vi "系统设置全局变量.vi"() -> ()   [LabVIEW 2016]
panel:
  in  "多参数运行间隔":i16=4 min=0 max=24
  in  "电源串口":refnum<visa-resource-name>
  out "流程测试中":bool
  out "24H周期设置":bool[](array[boolean])
  out "启用运维打卡":bool caption="启用"
  in  "权限密码":u32[](array[numeric])=[0, 23506, 783523506, 783523103]
  in  "站点系列号":string
  in  "系统重启设置":T1 {"分" max=59 format="%02.0f"; "时" max=23 format="%02.0f"}
  in  "首页显示信息设置":T2={"水温"=TRUE, "pH"=FALSE, "DO"=FALSE, "Cond"=FALSE, "Turb"=FALSE, "氨氮"=FALSE, "总磷"=FALSE, "总氮"=FALSE, "CODMn"=FALSE, "CODCr"=FALSE, "水位"=FALSE, "流速"=FALSE, "瞬时流量"=FALSE, "ORP"=FALSE, "氟化物"=FALSE, "铅"=FALSE, "镉"=FALSE, "铜"=FALSE, "锌"=FALSE, "汞"=FALSE, "叶绿素a"=FALSE, "藻密度"=FALSE, "氯化物"=FALSE, "挥发酚"=FALSE, "盐度"=FALSE}
  # "频次："
  # "时间："
  # "："
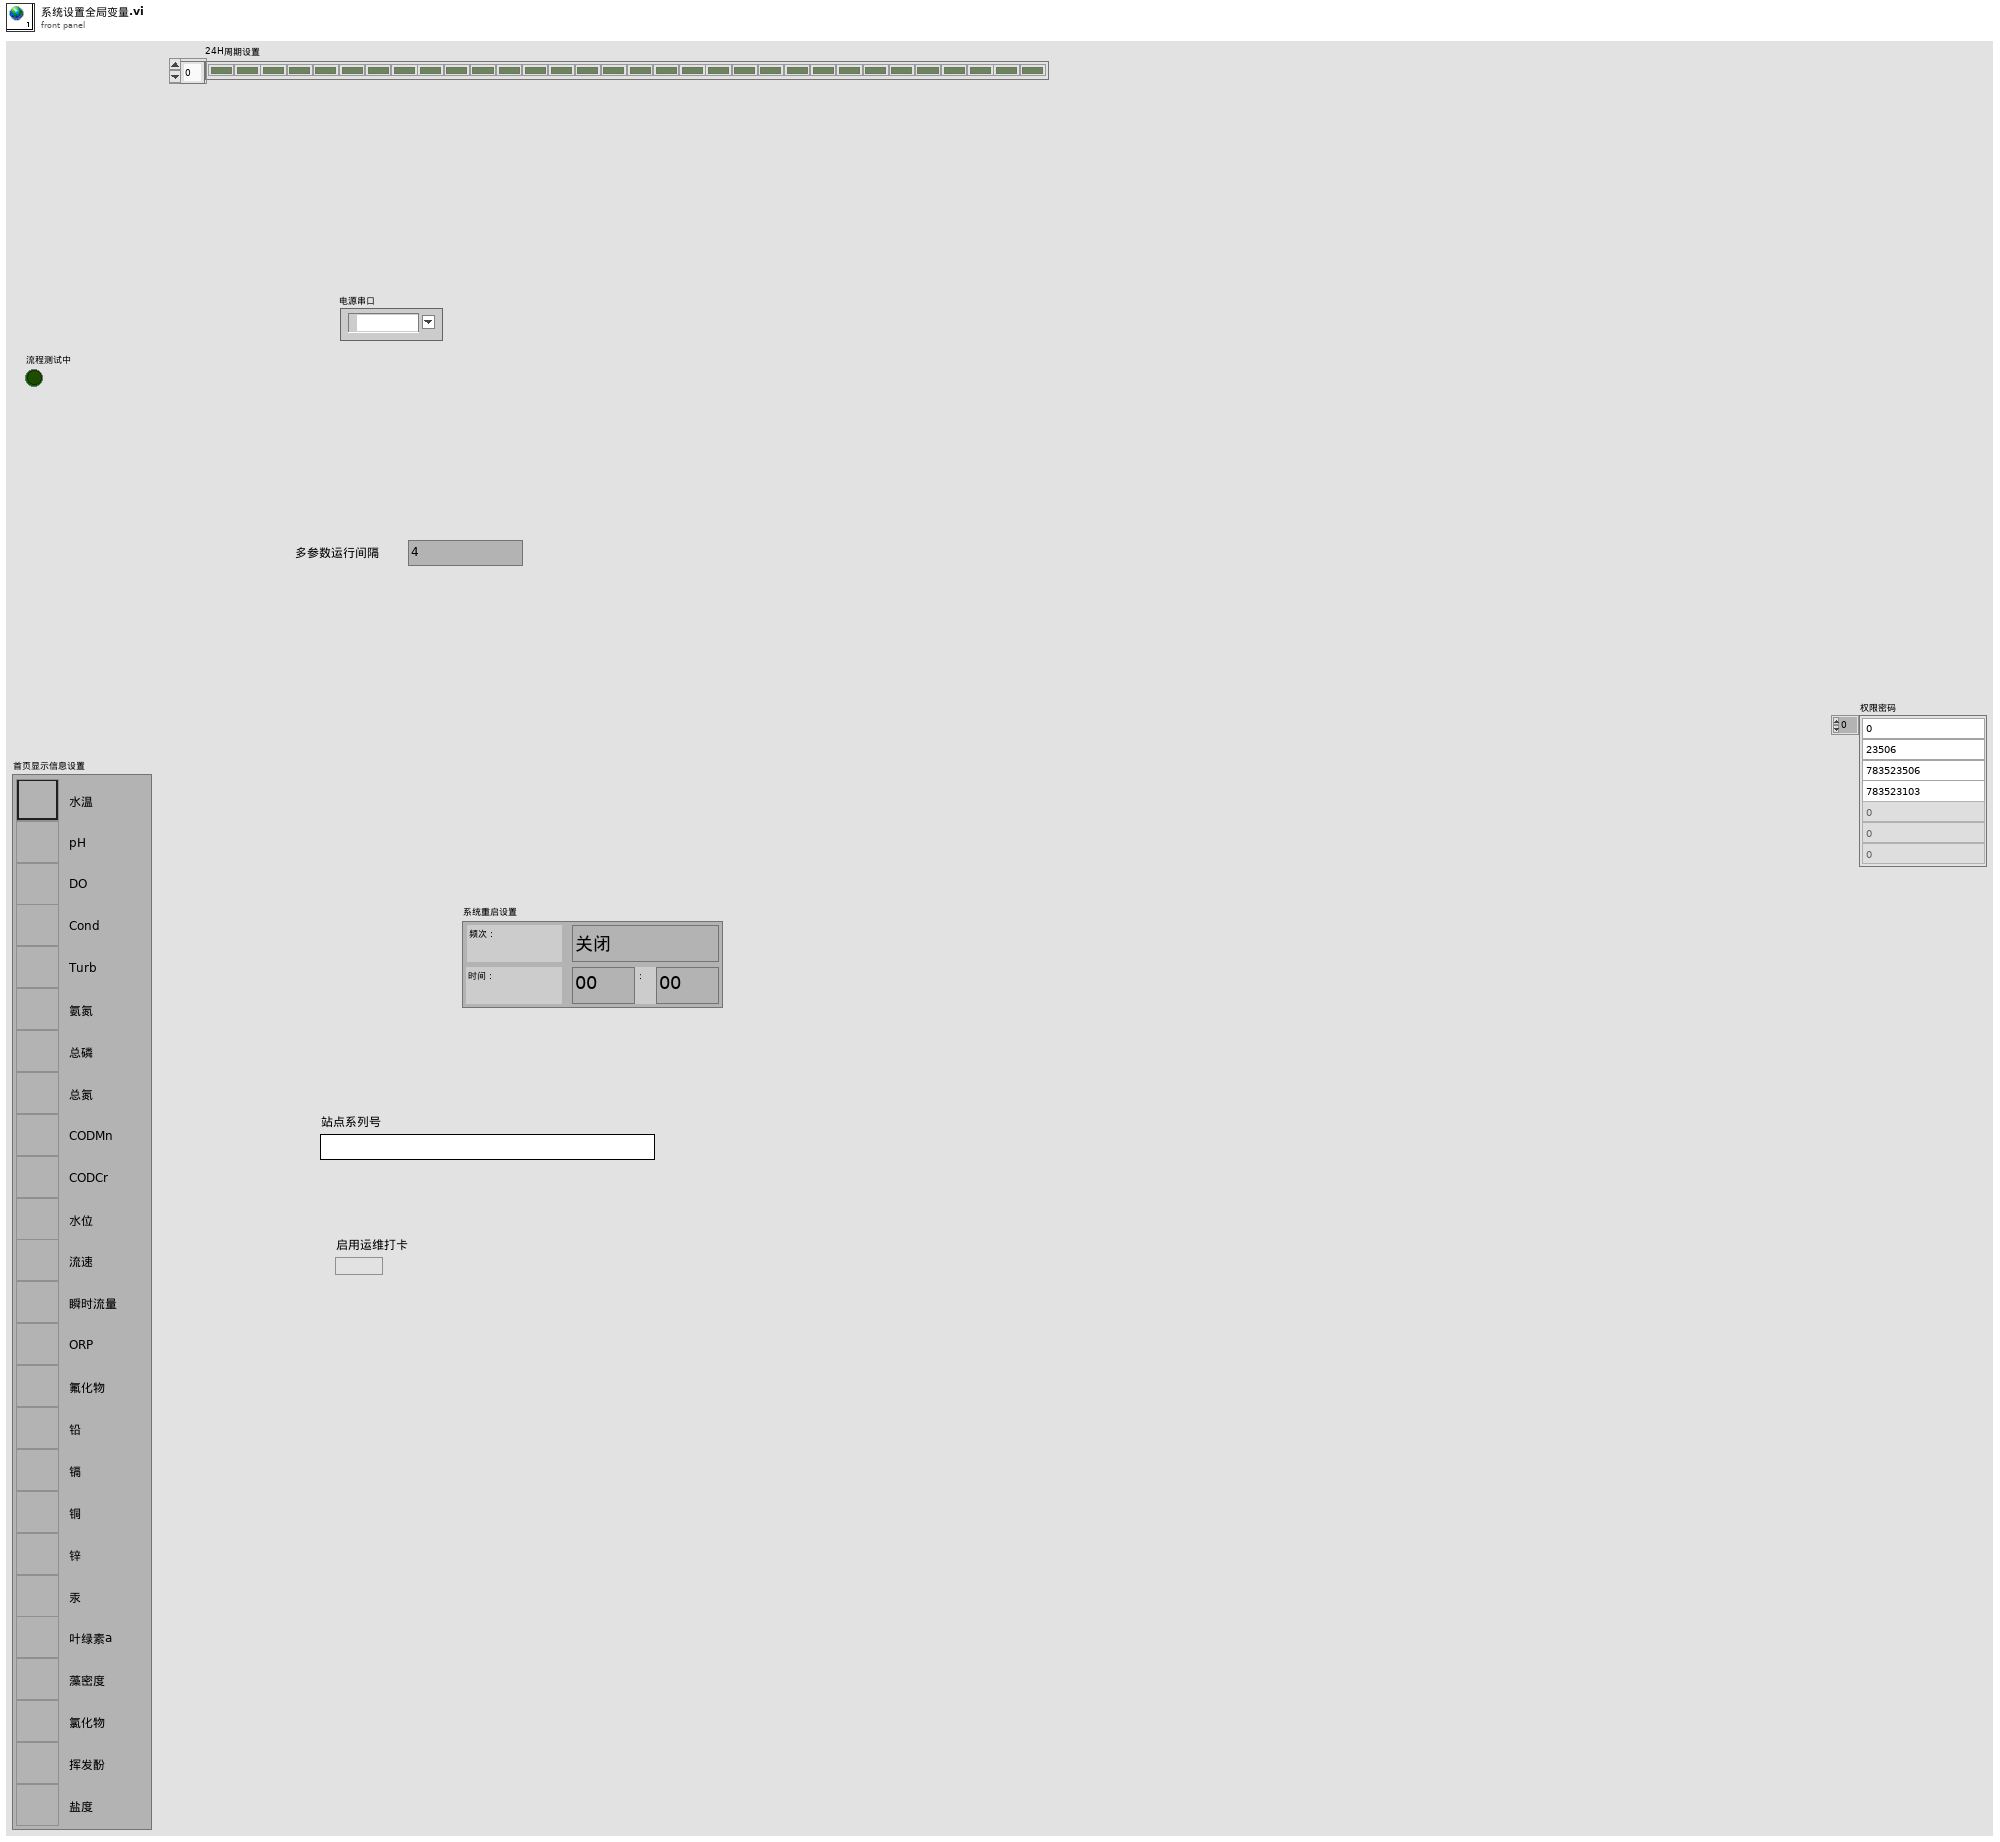
[diagram p1: front panel]
types:
  T1 = cluster{"频次":enum16{"关闭", "每天", "星期一", "星期二", "星期三", "星期四", "星期五", "星期六", "星期日"}, "时":u16, "分":u16}
  T2 = cluster{"水温":bool, "pH":bool, "DO":bool, "Cond":bool, "Turb":bool, "氨氮":bool, "总磷":bool, "总氮":bool, "CODMn":bool, "CODCr":bool, "水位":bool, "流速":bool, "瞬时流量":bool, "ORP":bool, "氟化物":bool, "铅":bool, "镉":bool, "铜":bool, "锌":bool, "汞":bool, "叶绿素a":bool, "藻密度":bool, "氯化物":bool, "挥发酚":bool, "盐度":bool}
diagram:
